vi "verify #cycles.vi"(8 "error in (no error)":errorcluster, 11 "Simulated Camera in":refnum<class "Sim_Ixon_Ultra.lvclass">) -> (0 "error out":errorcluster, 3 "Simulated Camera out":refnum<class "Sim_Ixon_Ultra.lvclass">)   [LabVIEW 2018, in "Sim_Ixon_Ultra.lvclass"]
uses:
  Sim_Ixon_Ultra.lvclass
  Sim_Ixon_Ultra.lvclass/Sim_Ixon_Ultra.ctl
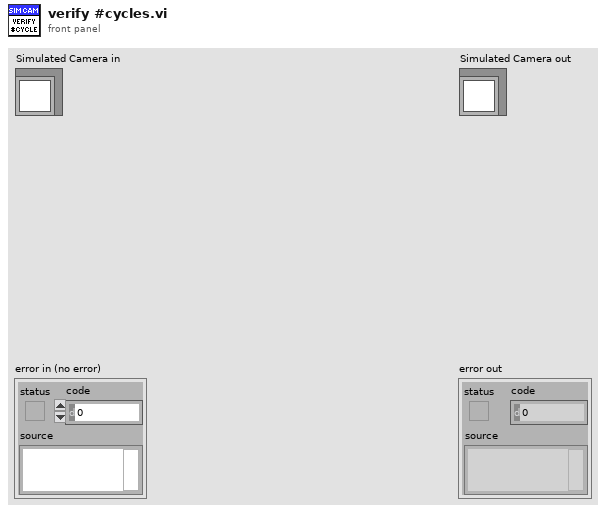
[diagram p1: front panel]
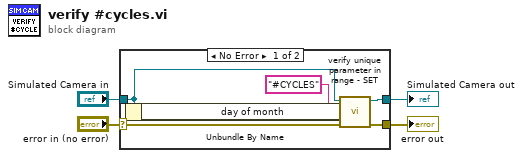
[diagram p0: block diagram]
diagram:
  n1 = case shown="No Error" "error in (no error)" {
    selector: "error in (no error)" -> [w10 w12]
    tunnel: [w9 w12] -> w3
    tunnel: [w8 w11] -> w1
    tunnel: "Simulated Camera in" -> [w6 w11]
    frame No Error {
      n2 = Unbundle By Name(w6) -> ("day of month"=w5:i32)
      n3 = call "verify unique parameter in range - SET.vi"("error in (no error)"=w10, "value"=w5, "parameter name"="#CYCLES", "Simulated_CCD_Camera in"=w6) -> ("error out"=w9:errorcluster, "Simulated_CCD_Camera out"=w8:refnum<class "Sim_Ixon_Ultra.lvclass">)  [unwired: 6 in]
    }
    frame Error {
    }
  }
  "error out" <- w3
  "Simulated Camera out" <- w1
